vi "DigitalIn_mode.vi"(8 "error in (no error)":errorcluster, 10 "PinMode":enum16{""}(ring), 11 "DigitalIn in":refnum<class "DigitalIn.lvclass">) -> (0 "error out":errorcluster, 3 "DigitalIn out":refnum<class "DigitalIn.lvclass">)   [LabVIEW 2011, in "mbed_LVLibrary.lvlib" / "DigitalIn.lvclass"]
uses:
  DigitalIn.lvclass
  DigitalIn.lvclass/DigitalIn.ctl
  Transport Mechanisms/mbed/mbed.lvclass
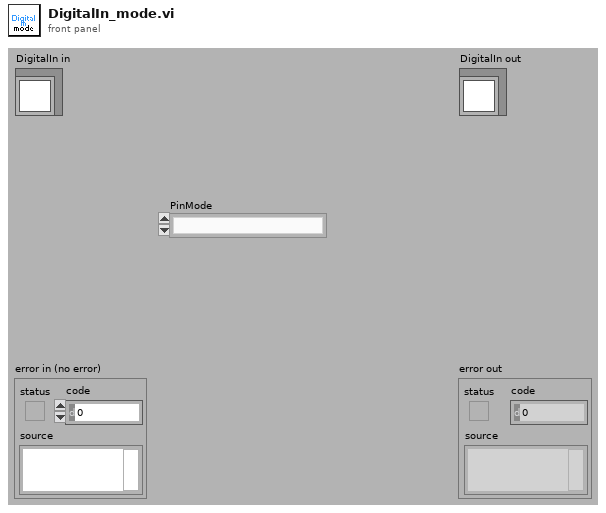
[diagram p1: front panel]
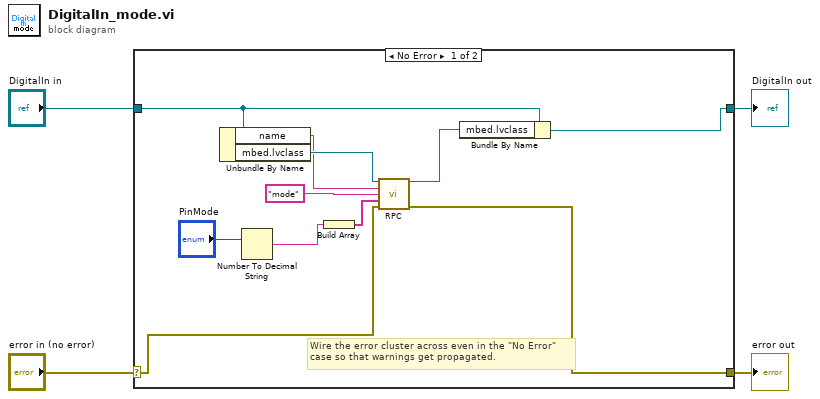
[diagram p0: block diagram]
diagram:
  n1 = case shown="No Error" "error in (no error)" {
    selector: "error in (no error)" -> [w6 w17]
    tunnel: [w5 w17] -> w3
    tunnel: [w8 w16] -> w1
    tunnel: "DigitalIn in" -> [w9 w16]
    frame No Error {
      # "Wire the error cluster across even in the \"No Error\"\ncase so that warnings get propagated."
      n2 = Unbundle By Name(w9) -> ("name"=w14:string, "mbed.lvclass"=w15:refnum<class "mbed.lvclass">)
      n3 = Number To Decimal String(number="PinMode") -> (decimal integer string=w11:string)  [unwired: 1 in]
      n4 = Build Array(w11) -> (w12:string[])
      n5 = call-dynamic "RPC.vi"("mbed in"=w15, "Name"=w14, "method"="mode", "Args"=w12, "error in (no error)"=w6) -> ("mbed out"=w7:refnum<class "mbed.lvclass">, "error out"=w5:errorcluster)  [unwired: 8 in, 1 out]
      n6 = Bundle By Name(cluster=w9, "mbed.lvclass"=w7) -> (w8:refnum<class "DigitalIn.lvclass">)
    }
    frame Error {
    }
  }
  "error out" <- w3
  "DigitalIn out" <- w1
